vi "Send Launch Nested.vi"(8 "error in (no error)":errorcluster, 9 "Config Element":refnum<class "VolatusConfigElement.lvclass">, 10 "Nested Module":refnum<class "Module.lvclass">, 11 "Module in":refnum<class "Module.lvclass">) -> (0 "error out":errorcluster, 3 "Module out":refnum<class "Module.lvclass">)   [LabVIEW 2020, in "Volatus.lvlib" / "Module.lvclass"]
uses:
  Module.lvclass
  VolatusConfig/VolatusConfigElement/VolatusConfigElement.lvclass
  Launch Nested Message.ctl
  Module.lvclass/Module.ctl
  MessageQ/MessageQ.lvclass/MessageQ.ctl
  Volatus.lvlib
  MessageQ/MessageQ.lvclass
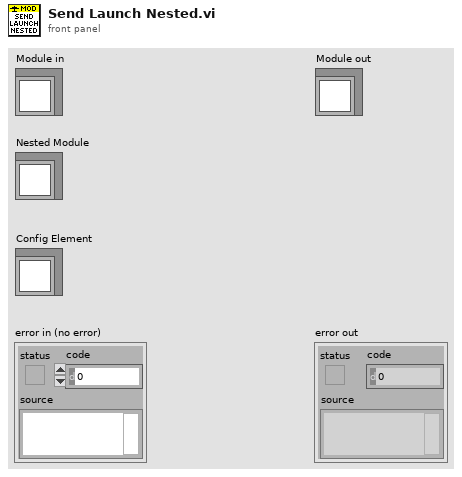
[diagram p1: front panel]
types:
  T1 = typedef "Volatus.lvlib/Launch Nested Message.ctl" = cluster{"Module":refnum<class "Module.lvclass">, "Config":refnum<class "VolatusConfigElement.lvclass">}
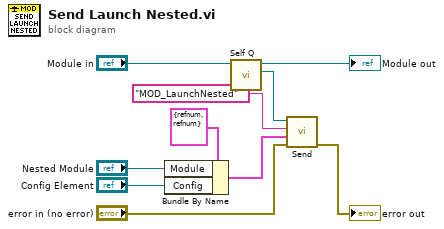
[diagram p0: block diagram]
diagram:
  n1 = Bundle By Name(cluster=T1 {"Module"=refnum, "Config"=refnum} ("Launch Nested Message"), "Module"="Nested Module", "Config"="Config Element") -> (w5:T1)
  n2 = call "Self Q.vi"("Module in"="Module in") -> ("Self Q"=w4:refnum<class "MessageQ.lvclass">, "Module out"=→"Module out":refnum<class "Module.lvclass">)  [unwired: 9 in]
  n3 = call "Send.vi"("error in (no error)"="error in (no error)", "Data"=w5, "ID"="MOD_LaunchNested", "MessageQ in"=w4) -> ("error out"=→"error out":errorcluster)  [unwired: 6 in, 1 out]
